vi "Get Position Piezo.vi"(5 "Piezo State":T2, 7 "Counter Time":i32, 8 "error in (no error)":errorcluster, 9 "notifier out":refnum<notifier>, 11 "Cluster":T1={"physical channels"="Dev5/ao0", "MAX   VOLTAGE"=10.0, "MIN   VOLTAGE"=0.0}) -> (0 "error out":errorcluster, 3 "Cluster 2":T1={"physical channels"="Dev5/ao0", "MAX   VOLTAGE"=10.0, "MIN   VOLTAGE"=0.0})   [LabVIEW 2013, in "Piezo.lvlib"]
uses:
  Piezo/Piezo.lvlib
  Piezo/Piezo State.ctl
  Piezo/Piezo display.ctl
  Untitled Project 3 Andrea/piezo new/Hardware Configuration Piezo out.ctl
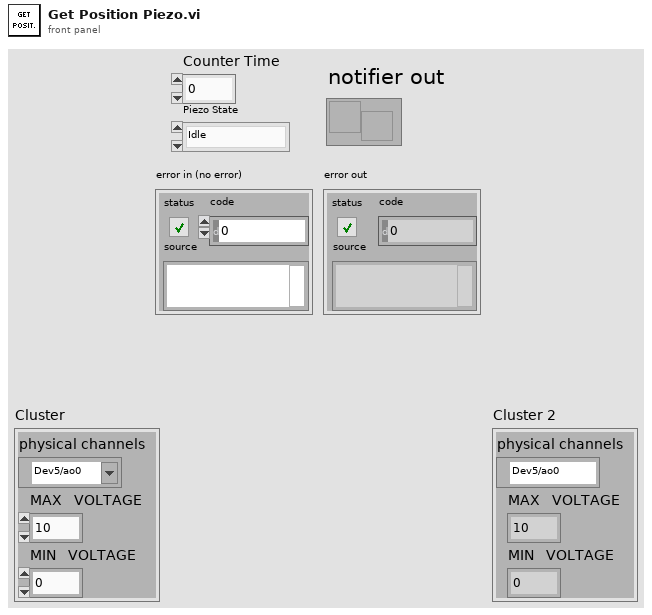
[diagram p1: front panel]
types:
  T1 = typedef "Hardware Configuration Piezo out.ctl" = cluster{"physical channels":tag, "MAX   VOLTAGE":dbl, "MIN   VOLTAGE":dbl}
  T2 = typedef "Piezo.lvlib/Piezo State.ctl" = enum16{"Idle", "Acquiring"}
  T3 = typedef "Piezo.lvlib/Piezo display.ctl" = cluster{"PiezoPosition":sgl, "Counter Time":i32}
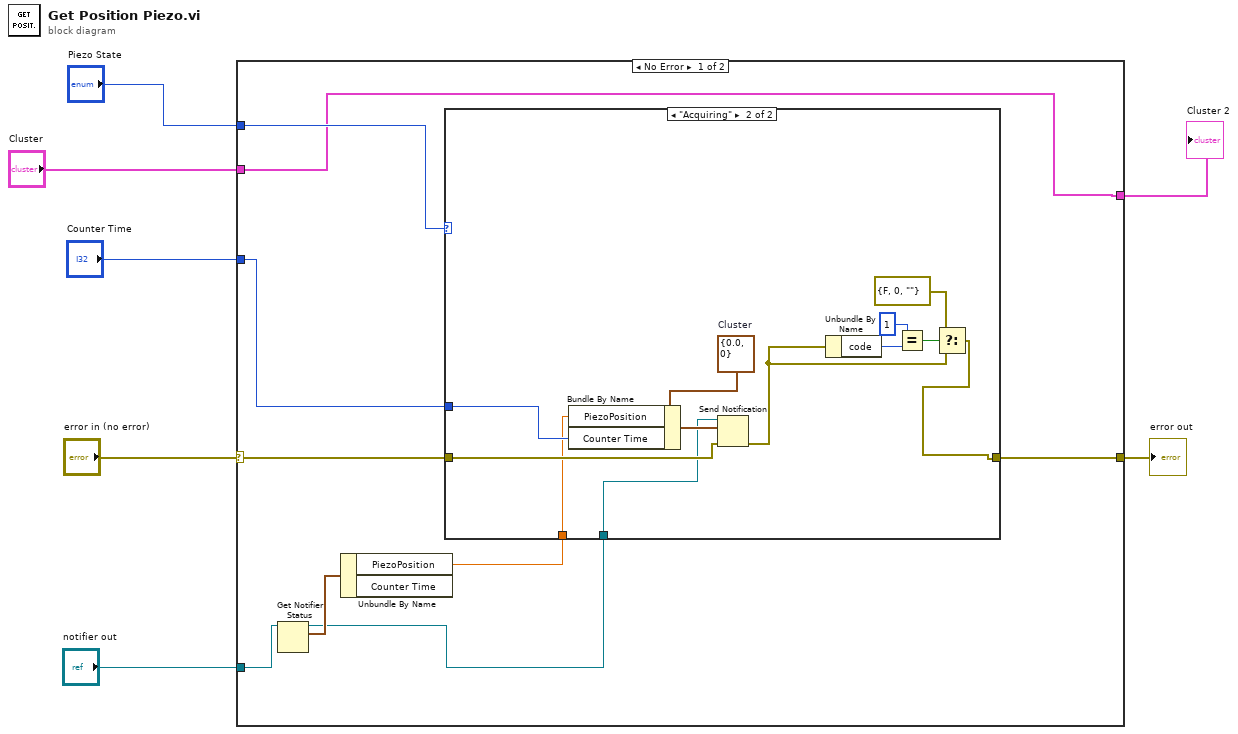
[diagram p0: block diagram]
diagram:
  n1 = case shown="No Error" "error in (no error)" {
    selector: "error in (no error)" -> [w14 w31]
    tunnel: [w13 w31] -> w6
    tunnel: "Piezo State" -> [w16 _]
    tunnel: "Counter Time" -> [w15 _]
    tunnel: "notifier out" -> [w11 _]
    tunnel: [w8 w30] -> w2
    tunnel: "Cluster" -> [w8 w30]
    frame No Error {
      n2 = Get Notifier Status(notifier=w11) -> (notifier out=w10:refnum<notifier>, current notification=w12:T3)  [unwired: 1 in, 3 out]
      n3 = Unbundle By Name(w12) -> ("PiezoPosition"=w9:sgl)  [unwired: 1 out]
      n4 = case shown="\"Acquiring\"" w16 {
        tunnel: w15 -> [_ w27]
        tunnel: w10 -> [_ w21]
        tunnel: w14 -> [w17 w28]
        tunnel: [w17 w18] -> w13
        tunnel: w9 -> [_ w19]
        frame "Idle", Default {
        }
        frame "Acquiring" {
          w26 = T3 {"PiezoPosition"=0.0, "Counter Time"=0}  # Cluster
          n5 = Bundle By Name(cluster=w26, "PiezoPosition"=w19, "Counter Time"=w27) -> (w29:T3)
          n6 = Send Notification(notification=w29, notifier=w21, error in (no error)=w28) -> (error out=w20:errorcluster)  [unwired: 1 out]
          n7 = Unbundle By Name(w20) -> ("code"=w25:i32)
          n8 = Equal?(x=1, y=w25) -> (x = y?=w23:bool)
          n9 = Select(t=errorcluster {"status"=FALSE, "code"=0, "source"=""} ("error constant"), s=w23, f=w20) -> (s? t:f=w18:errorcluster)
        }
      }
    }
    frame Error {
    }
  }
  "error out" <- w6
  "Cluster 2" <- w2
